vi "SetVoltage.vi"(8 "error in (no error)":errorcluster, 9 "Voltage":dbl, 10 "Channel":i8, 11 "TecellaClient in":refnum<class "TecellaClient.lvclass">) -> (0 "error out":errorcluster, 3 "TecellaClient out":refnum<class "TecellaClient.lvclass">)   [LabVIEW 2009, in "TecellaClient.lvclass"]
uses:
  TecellaClient.lvclass
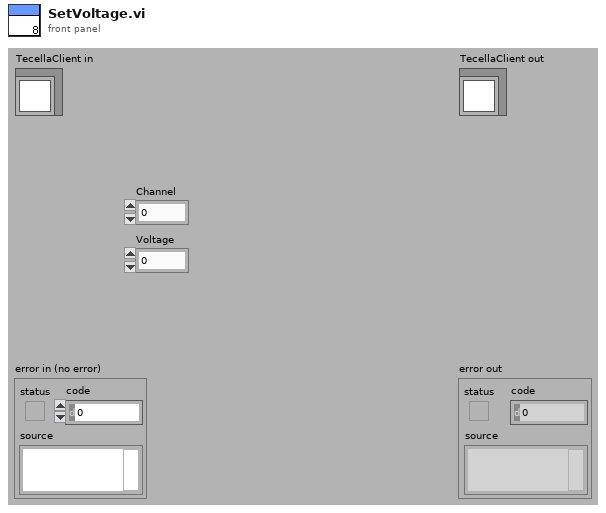
[diagram p1: front panel]
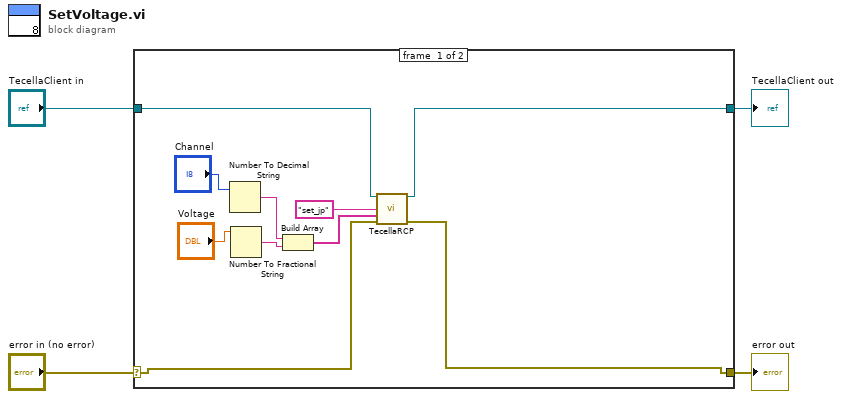
[diagram p0: block diagram]
diagram:
  n1 = case shown="No Error" "error in (no error)" {
    selector: "error in (no error)" -> [w12 w16]
    tunnel: [w11 w16] -> w3
    tunnel: [w13 w15] -> w1
    tunnel: "TecellaClient in" -> [w14 w15]
    frame #0 {
      n2 = Number To Decimal String(number="Channel") -> (decimal integer string=w5:string)  [unwired: 1 in]
      n3 = Number To Fractional String(number="Voltage") -> (F-format string=w7:string)  [unwired: 3 in]
      n4 = Build Array(w5, w7) -> (w9:string[])
      n5 = call-dynamic "TecellaRCP.vi"("TecellaClient in"=w14, "method"="set_jp", "Args"=w9, "error in (no error)"=w12) -> ("TecellaClient out"=w13:refnum<class "TecellaClient.lvclass">, "error out"=w11:errorcluster)  [unwired: 9 in, 1 out]
    }
    frame #1 {
    }
  }
  "error out" <- w3
  "TecellaClient out" <- w1
